vi "Get Value (Array).vi"(8 "error in (no error)":errorcluster, 10 "key":string, 11 "JSON Object in":refnum<class "JSON Object.lvclass">) -> (0 "error out":errorcluster, 2 "value":refnum<class "JSON Array.lvclass">)   [LabVIEW 2015, in "LVJSON.lvlib" / "JSON Object.lvclass"]
uses:
  JSON Object.lvclass
  JSON Array/JSON Array.lvclass
  JSON Helper/To More Specific Type (Array).vi
  JSON Helper/JSON Helper.lvclass
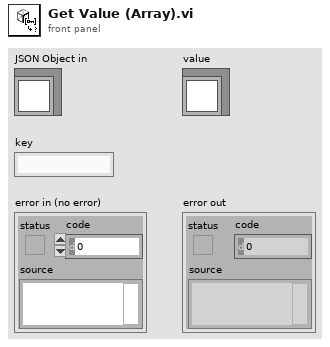
[diagram p1: front panel]
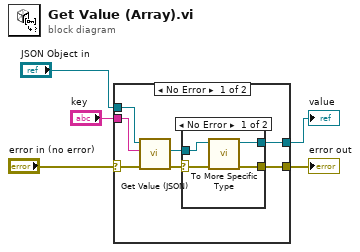
[diagram p0: block diagram]
diagram:
  n1 = case shown="No Error" "error in (no error)" {
    selector: "error in (no error)" -> [w10 w18]
    tunnel: [w7 w18] -> w4
    tunnel: "JSON Object in" -> [w12 _]
    tunnel: "key" -> [w11 _]
    tunnel: [w6 _] -> w1
    frame No Error {
      n2 = call "Get Value (JSON).vi"("error in (no error)"=w10, "key"=w11, "JSON Object in"=w12) -> ("error out"=w8:errorcluster, "value"=w9:refnum<class "JSON Null.lvclass">)  [unwired: 7 in]
      n3 = case shown="No Error" w8 {
        selector: w8 -> [w16 w17]
        tunnel: w9 -> [w13 _]
        tunnel: [w15 w17] -> w7
        tunnel: [w14 _] -> w6
        frame No Error {
          n4 = call-poly "To More Specific Type.vi"("error in (no error)"=w16, "JSON Datatype in"=w13) -> ("error out"=w15:errorcluster, "JSON Datatype out"=w14:refnum<class "JSON Array.lvclass">)  [unwired: 8 in]
        }
        frame Error {
        }
      }
    }
    frame Error {
    }
  }
  "error out" <- w4
  "value" <- w1
